vi "Convert CAN Trace to Raw Frame.vi"(8 "error in":errorcluster, 11 "captured data in":string[][](array[string])) -> (0 "error out":errorcluster, 2 "raw frames":u8[](array[numeric]) format="%02x")   [LabVIEW 2025, in "CAN-LIN Raw Bus Capture UI.lvlib"]
uses:
  CAN-LIN Raw Bus Capture UI.lvlib
  <vilib>/xnet/xnet.llb/XNET Frame CAN.ctl
  <vilib>/xnet/xnet.llb/XNET Frame Type CAN.ctl
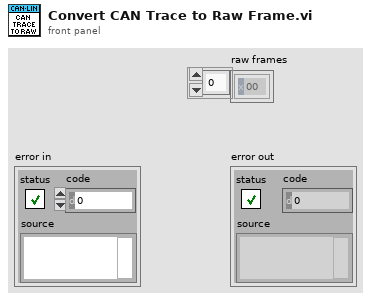
[diagram p1: front panel]
types:
  T1 = typedef "XNET Frame CAN.ctl" = cluster{"timestamp":timestamp, "payload":u8[], "identifier":u32, "type":T2, "extended?":bool, "echo?":bool}
  T2 = typedef "XNET Frame Type CAN.ctl" = u8
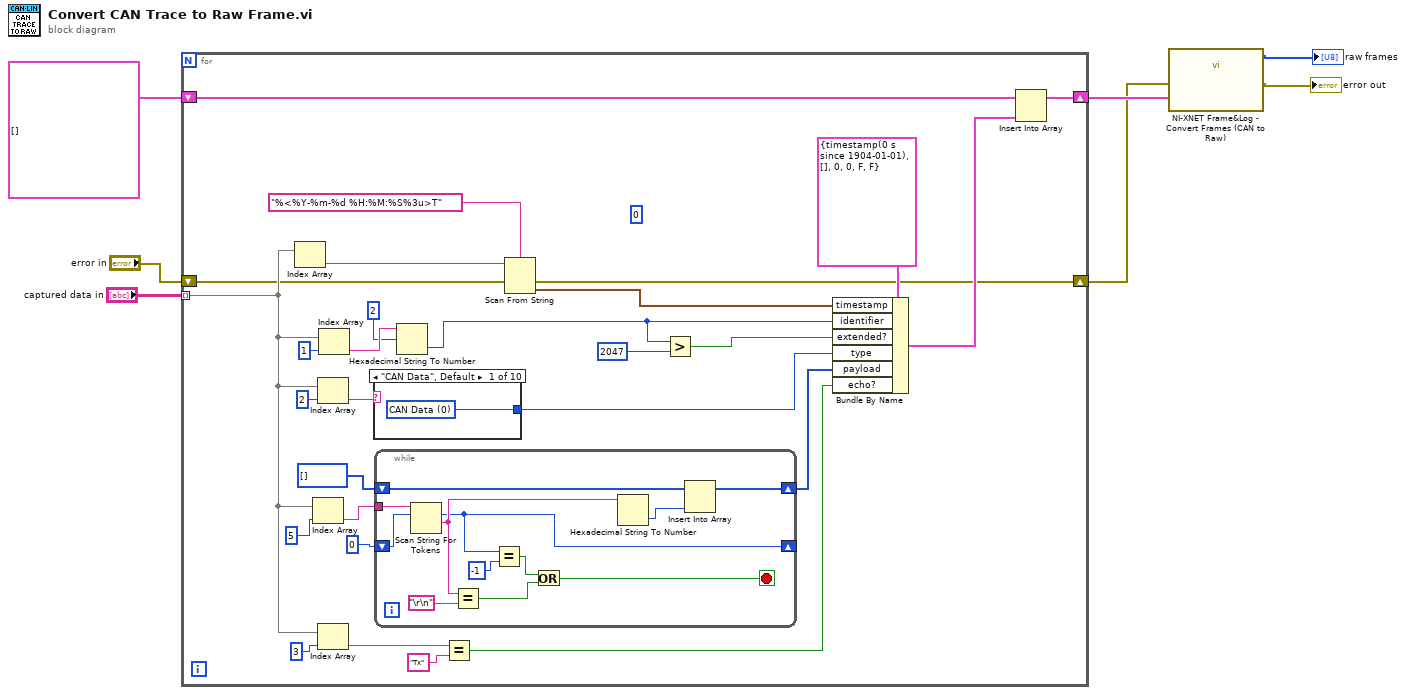
[diagram p0: block diagram]
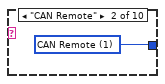
[diagram p2: hidden frame]
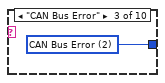
[diagram p3: hidden frame]
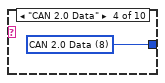
[diagram p4: hidden frame]
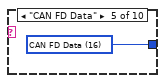
[diagram p5: hidden frame]
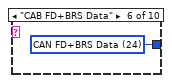
[diagram p6: hidden frame]
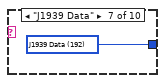
[diagram p7: hidden frame]
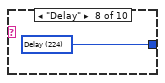
[diagram p8: hidden frame]
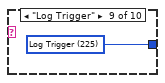
[diagram p9: hidden frame]
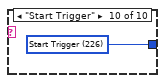
[diagram p10: hidden frame]
diagram:
  n1 = for {
    tunnel: "captured data in" -> [w20] mode=indexing
    shift-right: [w32] -> w5
    shift-left: T1[] [] ("CAN frames") -> [w33]
    shift-right: [w18] -> w1
    shift-left: "error in" -> [w11]
    (unwired) u32 0 ("number")
    n2 = Index Array(array=w20) -> (element=w10:string)  [unwired: 1 in]
    n3 = Index Array(array=w20, index=5) -> (element=w25:string)
    n4 = Index Array(array=w20, index=2) -> (element=w27:string)
    n5 = Index Array(array=w20, index=3) -> (element=w22:string)
    n6 = Index Array(array=w20, index=1) -> (element=w29:string)
    n7 = case shown="\"CAN Data\", Default" w27 {
      tunnel: [w48 w49 w50 w51 w52 w53 w54 w55 w56 w57] -> w14
      frame "CAN Data", Default {
        w48 = T2 0 items=["CAN Data"=0, "CAN Remote"=1, "CAN Bus Error"=2, "CAN 2.0 Data"=8, "CAN FD Data"=16, "CAN FD+BRS Data"=24, "J1939 Data"=192, "Delay"=224, "Log Trigger"=225, "Start Trigger"=226] ("type")
      }
      frame "CAN Remote" {
        w49 = T2 1 items=["CAN Data"=0, "CAN Remote"=1, "CAN Bus Error"=2, "CAN 2.0 Data"=8, "CAN FD Data"=16, "CAN FD+BRS Data"=24, "J1939 Data"=192, "Delay"=224, "Log Trigger"=225, "Start Trigger"=226] ("type")
      }
      frame "CAN Bus Error" {
        w50 = T2 2 items=["CAN Data"=0, "CAN Remote"=1, "CAN Bus Error"=2, "CAN 2.0 Data"=8, "CAN FD Data"=16, "CAN FD+BRS Data"=24, "J1939 Data"=192, "Delay"=224, "Log Trigger"=225, "Start Trigger"=226] ("type")
      }
      frame "CAN 2.0 Data" {
        w51 = T2 8 items=["CAN Data"=0, "CAN Remote"=1, "CAN Bus Error"=2, "CAN 2.0 Data"=8, "CAN FD Data"=16, "CAN FD+BRS Data"=24, "J1939 Data"=192, "Delay"=224, "Log Trigger"=225, "Start Trigger"=226] ("type")
      }
      frame "CAN FD Data" {
        w52 = T2 16 items=["CAN Data"=0, "CAN Remote"=1, "CAN Bus Error"=2, "CAN 2.0 Data"=8, "CAN FD Data"=16, "CAN FD+BRS Data"=24, "J1939 Data"=192, "Delay"=224, "Log Trigger"=225, "Start Trigger"=226] ("type")
      }
      frame "CAB FD+BRS Data" {
        w53 = T2 24 items=["CAN Data"=0, "CAN Remote"=1, "CAN Bus Error"=2, "CAN 2.0 Data"=8, "CAN FD Data"=16, "CAN FD+BRS Data"=24, "J1939 Data"=192, "Delay"=224, "Log Trigger"=225, "Start Trigger"=226] ("type")
      }
      frame "J1939 Data" {
        w54 = T2 192 items=["CAN Data"=0, "CAN Remote"=1, "CAN Bus Error"=2, "CAN 2.0 Data"=8, "CAN FD Data"=16, "CAN FD+BRS Data"=24, "J1939 Data"=192, "Delay"=224, "Log Trigger"=225, "Start Trigger"=226] ("type")
      }
      frame "Delay" {
        w55 = T2 224 items=["CAN Data"=0, "CAN Remote"=1, "CAN Bus Error"=2, "CAN 2.0 Data"=8, "CAN FD Data"=16, "CAN FD+BRS Data"=24, "J1939 Data"=192, "Delay"=224, "Log Trigger"=225, "Start Trigger"=226] ("type")
      }
      frame "Log Trigger" {
        w56 = T2 225 items=["CAN Data"=0, "CAN Remote"=1, "CAN Bus Error"=2, "CAN 2.0 Data"=8, "CAN FD Data"=16, "CAN FD+BRS Data"=24, "J1939 Data"=192, "Delay"=224, "Log Trigger"=225, "Start Trigger"=226] ("type")
      }
      frame "Start Trigger" {
        w57 = T2 226 items=["CAN Data"=0, "CAN Remote"=1, "CAN Bus Error"=2, "CAN 2.0 Data"=8, "CAN FD Data"=16, "CAN FD+BRS Data"=24, "J1939 Data"=192, "Delay"=224, "Log Trigger"=225, "Start Trigger"=226] ("type")
      }
    }
    n8 = while {
      tunnel: w25 -> [w47]
      shift-right: [w36] -> w15
      shift-left: u8[] [] ("payload") -> [w45]
      shift-right: [w39] -> _
      shift-left: 0 ("offset") -> [w43]
      stop <- w42 stop-if-true
      n9 = Scan String For Tokens(8:w43, 9:w47) -> (1:w44:string, 2:w39:i32)  [unwired: 4 in, 2 out]
      n10 = Equal?(x=w44, y="\r\n") -> (x = y?=w41:bool)
      n11 = Equal?(x=w39, y=-1) -> (x = y?=w40:bool)
      n12 = Or(x=w40, y=w41) -> (x .or. y?=w42:bool)
      n13 = Hexadecimal String To Number(string=w44) -> (number=w37:u32)  [unwired: 2 in, 1 out]
      n14 = Insert Into Array(array=w45, new element=w37) -> (w36:u8[])  [unwired: 1 in]
    }
    n15 = Hexadecimal String To Number(string=w29, offset=2) -> (number=w9:u32)  [unwired: 1 in, 1 out]
    n16 = Equal?(x=w22, y="Tx") -> (x = y?=w16:bool)
    n17 = Scan From String(format string="%<%Y-%m-%d %H:%M:%S%3u>T", input string=w10, error in=w11) -> (error out=w18:errorcluster, output 1=w31:timestamp)  [unwired: 2 in, 2 out]
    n18 = Greater?(x=w9, y=u32 2047) -> (0:w13:bool)
    n19 = Bundle By Name(cluster=T1 {"timestamp"=timestamp(0 s since 1904-01-01), "payload"=[], "identifier"=0, "type"=0, "extended?"=FALSE, "echo?"=FALSE} ("CAN frame"), "timestamp"=w31, "identifier"=w9, "extended?"=w13, "type"=w14, "payload"=w15, "echo?"=w16) -> (w34:T1)
    n20 = Insert Into Array(array=w33, new element=w34) -> (w32:T1[])  [unwired: 1 in]
  }
  n21 = call "NI-XNET Frame&Log - Convert Frames (CAN to Raw).vi"("CAN frames"=w5, "error in"=w1) -> ("raw frames"=→"raw frames":u8[], "error out"=→"error out":errorcluster)  [unwired: 11 in, 1 out]
